vi "Global_Instr.vi"() -> ()   [LabVIEW 2015]
panel:
  in  "Cluster":T1
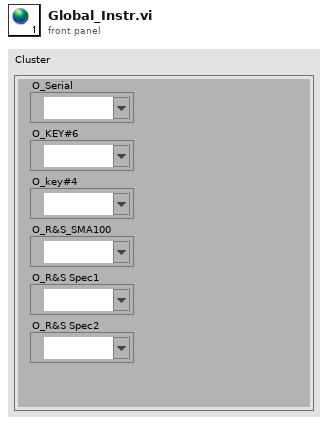
[diagram p1: front panel]
types:
  T1 = cluster{"O_Serial":refnum<visa-resource-name>, "O_KEY#6":refnum<visa-resource-name>, "O_key#4":refnum<visa-resource-name>, "O_R&S_SMA100":refnum<visa-resource-name>, "O_R&S Spec1":refnum<visa-resource-name>, "O_R&S Spec2":refnum<visa-resource-name>}
diagram:
